vi "test-translation2d.vi"() -> ()   [LabVIEW 2019]
uses:
  <vilib>/Rock Robotics/WPI/ThirdParty/JAS_Junk/TrajLib/Util_CalcDist.vi
  <vilib>/Rock Robotics/WPI/ThirdParty/JAS_Junk/TrajLib/Trajectory_Library.lvlib
  <vilib>/Rock Robotics/WPI/ThirdParty/JAS_Junk/TrajLib/TRANSLATION2D.ctl
panel:
  out "T10 X-7.79, Y=4.5":T1 {"Y" format="%14.3f"; "X" format="%14.3f"}
  out "T7 -- y -- 0":dbl
  out "T7 -- X -- 0":dbl
  out "T6 -- dist - 0":dbl
  out "T5 -- norm - 0":dbl
  out "T4 -- y -- 0":dbl
  out "T4 -- X -- 0":dbl
  out "T3 -- y -- 0":dbl
  out "T3 -- X -- 0":dbl
  out "T2 -- y -- 0":dbl
  out "T2 -- X -- 0":dbl
  out "T9 - False":bool
  out "T8 - True":bool
  out "T1 -- y -- 0":dbl
  out "T1 -- X -- 0":dbl
  out "T0 -- y -- 0":dbl
  out "T0 -- X -- 0":dbl
  # "Translation2D Test"
  # "Didn't implement divide"
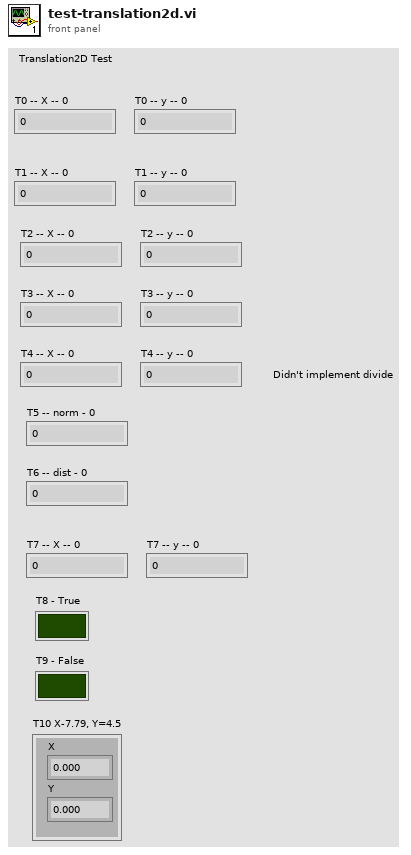
[diagram p1: front panel]
types:
  T1 = typedef "Trajectory_Library.lvlib/TRANSLATION2D.ctl" = cluster{"X":dbl, "Y":dbl}
  T2 = typedef "Trajectory_Library.lvlib/ROTATION2D.ctl" = cluster{"VALUE":dbl, "COS":dbl, "SIN":dbl}
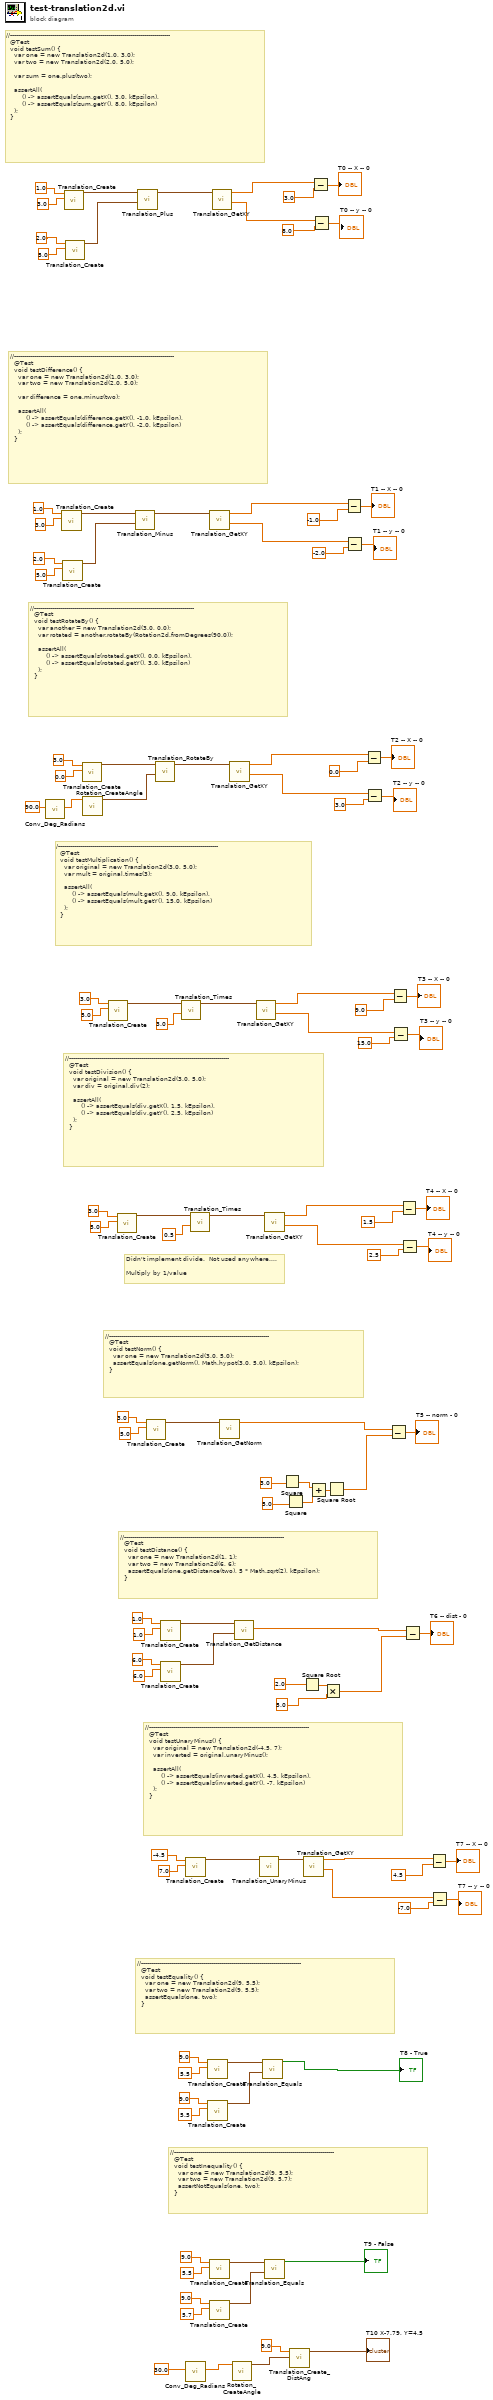
[diagram p0: block diagram]
diagram:
  # "//--------------------------------------------------------------------------------\n  @Test\n  void testInequality() {\n    var one = new Translation2d(9, 5.5);\n    var two = new Translation2d(9, 5.7);\n    assertNotEquals(one, two);\n  }"
  # "//--------------------------------------------------------------------------------\n  @Test\n  void testUnaryMinus() {\n    var original = new Translation2d(-4.5, 7);\n    var inverted = original.unaryMinus();\n\n    assertAll(\n        () -> assertEquals(inverted.getX(), 4.5, kEpsilon),\n        () -> assertEquals(inverted.getY(), -7, kEpsilon)\n    );\n  }"
  # "//--------------------------------------------------------------------------------\n  @Test\n  void testDistance() {\n    var one = new Translation2d(1, 1);\n    var two = new Translation2d(6, 6);\n    assertEquals(one.getDistance(two), 5 * Math.sqrt(2), kEpsilon);\n  }"
  # "//--------------------------------------------------------------------------------\n  @Test\n  void testNorm() {\n    var one = new Translation2d(3.0, 5.0);\n    assertEquals(one.getNorm(), Math.hypot(3.0, 5.0), kEpsilon);\n  }"
  # "Didn't implement divide.  Not used anywhere....\n\nMultiply by 1/value"
  # "//--------------------------------------------------------------------------------\n  @Test\n  void testDivision() {\n    var original = new Translation2d(3.0, 5.0);\n    var div = original.div(2);\n\n    assertAll(\n        () -> assertEquals(div.getX(), 1.5, kEpsilon),\n        () -> assertEquals(div.getY(), 2.5, kEpsilon)\n    );\n  }"
  # "/--------------------------------------------------------------------------------\n  @Test\n  void testMultiplication() {\n    var original = new Translation2d(3.0, 5.0);\n    var mult = original.times(3);\n\n    assertAll(\n        () -> assertEquals(mult.getX(), 9.0, kEpsilon),\n        () -> assertEquals(mult.getY(), 15.0, kEpsilon)\n    );\n  }"
  # "//--------------------------------------------------------------------------------\n  @Test\n  void testRotateBy() {\n    var another = new Translation2d(3.0, 0.0);\n    var rotated = another.rotateBy(Rotation2d.fromDegrees(90.0));\n\n    assertAll(\n        () -> assertEquals(rotated.getX(), 0.0, kEpsilon),\n        () -> assertEquals(rotated.getY(), 3.0, kEpsilon)\n    );\n  }"
  # "//--------------------------------------------------------------------------------\n  @Test\n  void testEquality() {\n    var one = new Translation2d(9, 5.5);\n    var two = new Translation2d(9, 5.5);\n    assertEquals(one, two);\n  }"
  # "//--------------------------------------------------------------------------------\n  @Test\n  void testDifference() {\n    var one = new Translation2d(1.0, 3.0);\n    var two = new Translation2d(2.0, 5.0);\n\n    var difference = one.minus(two);\n\n    assertAll(\n        () -> assertEquals(difference.getX(), -1.0, kEpsilon),\n        () -> assertEquals(difference.getY(), -2.0, kEpsilon)\n    );\n  }"
  # "//--------------------------------------------------------------------------------\n  @Test\n  void testSum() {\n    var one = new Translation2d(1.0, 3.0);\n    var two = new Translation2d(2.0, 5.0);\n\n    var sum = one.plus(two);\n\n    assertAll(\n        () -> assertEquals(sum.getX(), 3.0, kEpsilon),\n        () -> assertEquals(sum.getY(), 8.0, kEpsilon)\n    );\n  }"
  n1 = call <vilib>:"Conv_Deg_Radians.vi"("Degress"=90.0) -> ("Radians"=w77:dbl)  [unwired: 10 in]
  n2 = call <vilib>:"Translation_Create.vi"("Y"=3.0, "X"=1.0) -> ("TRANSLATION"=w93:T1)  [unwired: 9 in]
  n3 = call <vilib>:"Translation_Create.vi"("Y"=5.0, "X"=2.0) -> ("TRANSLATION"=w92:T1)  [unwired: 9 in]
  n4 = call <vilib>:"Translation_Create.vi"("Y"=3.0, "X"=1.0) -> ("TRANSLATION"=w102:T1)  [unwired: 9 in]
  n5 = call <vilib>:"Translation_Create.vi"("Y"=5.0, "X"=2.0) -> ("TRANSLATION"=w101:T1)  [unwired: 9 in]
  n6 = call <vilib>:"Translation_Create.vi"("Y"=0.0, "X"=3.0) -> ("TRANSLATION"=w82:T1)  [unwired: 9 in]
  n7 = call <vilib>:"Rotation_CreateAngle.vi"("Angle"=w77) -> ("ROTATION"=w75:T2)  [unwired: 10 in]
  n8 = call <vilib>:"Translation_Create.vi"("Y"=5.0, "X"=3.0) -> ("TRANSLATION"=w69:T1)  [unwired: 9 in]
  n9 = call <vilib>:"Translation_Create.vi"("Y"=5.0, "X"=3.0) -> ("TRANSLATION"=w58:T1)  [unwired: 9 in]
  n10 = call <vilib>:"Translation_Minus.vi"("other Translation"=w92, "In Translation"=w93) -> ("Out Translation"=w91:T1)  [unwired: 9 in]
  n11 = call <vilib>:"Translation_Plus.vi"("other Translation"=w101, "In Translation"=w102) -> ("Out Translation"=w100:T1)  [unwired: 9 in]
  n12 = call <vilib>:"Translation_Create.vi"("Y"=5.0, "X"=3.0) -> ("TRANSLATION"=w49:T1)  [unwired: 9 in]
  n13 = call <vilib>:"Translation_RotateBy.vi"("other Rotation"=w75, "In Translation"=w82) -> ("Out Translation"=w81:T1)  [unwired: 9 in]
  n14 = call <vilib>:"Translation_Create.vi"("Y"=1.0, "X"=1.0) -> ("TRANSLATION"=w38:T1)  [unwired: 9 in]
  n15 = call <vilib>:"Translation_Create.vi"("Y"=6.0, "X"=6.0) -> ("TRANSLATION"=w34:T1)  [unwired: 9 in]
  n16 = call <vilib>:"Translation_Times.vi"("Scalar"=3.0, "In Translation"=w69) -> ("Out Translation"=w68:T1)  [unwired: 9 in]
  n17 = call <vilib>:"Translation_Create.vi"("Y"=7.0, "X"=-4.5) -> ("TRANSLATION"=w27:T1)  [unwired: 9 in]
  n18 = call <vilib>:"Conv_Deg_Radians.vi"("Degress"=30.0 ("Y")) -> ("Radians"=w3:dbl)  [unwired: 10 in]
  n19 = call <vilib>:"Translation_Times.vi"("Scalar"=0.5, "In Translation"=w58) -> ("Out Translation"=w57:T1)  [unwired: 9 in]
  n20 = call <vilib>:"Translation_Create.vi"("Y"=5.5, "X"=9.0) -> ("TRANSLATION"=w14:T1)  [unwired: 9 in]
  n21 = call <vilib>:"Translation_Create.vi"("Y"=5.5, "X"=9.0) -> ("TRANSLATION"=w13:T1)  [unwired: 9 in]
  n22 = call <vilib>:"Translation_GetXY.vi"("In Translation"=w91) -> ("Y"=w89:dbl, "X"=w90:dbl)  [unwired: 9 in]
  n23 = call <vilib>:"Translation_Create.vi"("Y"=5.5, "X"=9.0) -> ("TRANSLATION"=w8:T1)  [unwired: 9 in]
  n24 = call <vilib>:"Translation_Create.vi"("Y"=5.7, "X"=9.0) -> ("TRANSLATION"=w7:T1)  [unwired: 9 in]
  n25 = call <vilib>:"Translation_GetXY.vi"("In Translation"=w100) -> ("Y"=w106:dbl, "X"=w107:dbl)  [unwired: 9 in]
  n26 = call <vilib>:"Translation_GetNorm.vi"("In Translation"=w49) -> ("Norm"=w43:dbl)  [unwired: 10 in]
  n27 = call <vilib>:"Translation_GetXY.vi"("In Translation"=w81) -> ("Y"=w79:dbl, "X"=w80:dbl)  [unwired: 9 in]
  n28 = call <vilib>:"Rotation_CreateAngle.vi"("Angle"=w3) -> ("ROTATION"=w4:T2)  [unwired: 10 in]
  n29 = call <vilib>:"Translation_GetDistance.vi"("other Translation"=w34, "In Translation"=w38) -> ("Distance"=w37:dbl)  [unwired: 9 in]
  n30 = call <vilib>:"Translation_GetXY.vi"("In Translation"=w68) -> ("Y"=w66:dbl, "X"=w67:dbl)  [unwired: 9 in]
  n31 = call <vilib>:"Translation_UnaryMinus.vi"("In Translation"=w27) -> ("Out Translation"=w22:T1)  [unwired: 10 in]
  n32 = call <vilib>:"Translation_Equals.vi"("other Translation"=w13, "In Translation"=w14) -> ("Equals"=→"T8 - True":bool)  [unwired: 9 in]
  n33 = call <vilib>:"Translation_GetXY.vi"("In Translation"=w57) -> ("Y"=w55:dbl, "X"=w56:dbl)  [unwired: 9 in]
  n34 = call <vilib>:"Translation_Equals.vi"("other Translation"=w7, "In Translation"=w8) -> ("Equals"=→"T9 - False":bool)  [unwired: 9 in]
  n35 = Square(x=3.0 ("X")) -> (x^2=w45:dbl)
  n36 = Square(x=5.0 ("X")) -> (x^2=w44:dbl)
  n37 = call <vilib>:"Translation_Create_DistAng.vi"("Angle"=w4, "Dist"=9.0 ("X")) -> ("TRANSLATION"=→"T10 X-7.79, Y=4.5":T1)  [unwired: 9 in]
  n38 = Square Root(x=2.0 ("X")) -> (sqrt(x)=w32:dbl)
  n39 = call <vilib>:"Translation_GetXY.vi"("In Translation"=w22) -> ("Y"=w20:dbl, "X"=w21:dbl)  [unwired: 9 in]
  n40 = Add(x=w45, y=w44) -> (x+y=w46:dbl)
  n41 = Subtract(x=w107, y=3.0) -> (x-y=→"T0 -- X -- 0":dbl)
  n42 = Subtract(x=w106, y=8.0) -> (x-y=→"T0 -- y -- 0":dbl)
  n43 = Multiply(x=w32, y=5.0 ("X")) -> (x*y=w30:dbl)
  n44 = Square Root(x=w46) -> (sqrt(x)=w42:dbl)
  n45 = Subtract(x=w90, y=-1.0 ("x")) -> (x-y=→"T1 -- X -- 0":dbl)
  n46 = Subtract(x=w89, y=-2.0) -> (x-y=→"T1 -- y -- 0":dbl)
  n47 = Subtract(x=w80, y=0.0 ("x")) -> (x-y=→"T2 -- X -- 0":dbl)
  n48 = Subtract(x=w79, y=3.0) -> (x-y=→"T2 -- y -- 0":dbl)
  n49 = Subtract(x=w43, y=w42) -> (x-y=→"T5 -- norm - 0":dbl)
  n50 = Subtract(x=w67, y=9.0 ("x")) -> (x-y=→"T3 -- X -- 0":dbl)
  n51 = Subtract(x=w66, y=15.0) -> (x-y=→"T3 -- y -- 0":dbl)
  n52 = Subtract(x=w56, y=1.5 ("x")) -> (x-y=→"T4 -- X -- 0":dbl)
  n53 = Subtract(x=w55, y=2.5) -> (x-y=→"T4 -- y -- 0":dbl)
  n54 = Subtract(x=w37, y=w30) -> (x-y=→"T6 -- dist - 0":dbl)
  n55 = Subtract(x=w21, y=4.5 ("x")) -> (x-y=→"T7 -- X -- 0":dbl)
  n56 = Subtract(x=w20, y=-7.0) -> (x-y=→"T7 -- y -- 0":dbl)
